vi "FIT line pad length.vi"(8 "error in":errorcluster, 11 "file (use dialog)":path) -> (0 "error out":errorcluster, 3 "FITS hdr":string[](array[string]))   [LabVIEW 2020]
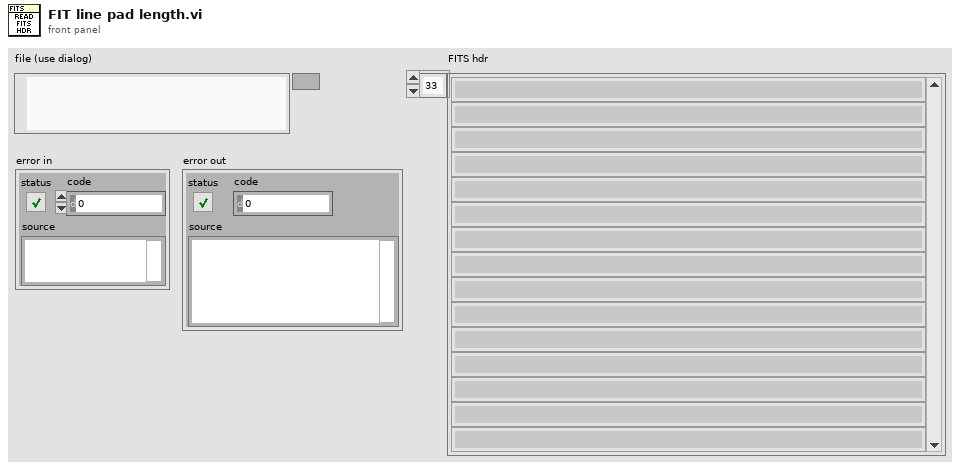
[diagram p1: front panel]
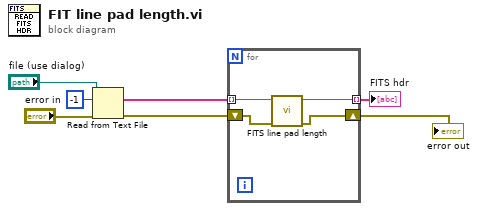
[diagram p0: block diagram]
diagram:
  n1 = Read from Text File(file (use dialog)="file (use dialog)", count=-1, error in="error in") -> (text=w5:string[], error out=w2:errorcluster)  [unwired: 1 in, 2 out]
  n2 = for {
    tunnel: w5 -> [w11] mode=indexing
    tunnel: [w10] -> w4 mode=indexing
    shift-right: [w8] -> w1
    shift-left: w2 -> [w9]
    n3 = call "FITS line pad length.vi"("error in (no error)"=w9, "Line"=w11) -> ("error out"=w8:errorcluster, "Padded Line"=w10:string)  [unwired: 8 in]
  }
  "FITS hdr" <- w4
  "error out" <- w1
